vi "Settings Poly.vi"   [LabVIEW 2011]
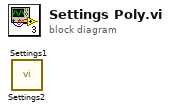
[diagram p0: block diagram]
diagram:
  n1 = call "Settings2.vi"() -> ()  [unwired: 11 in, 1 out]
  n2 = call "Settings1.vi"() -> ()  [unwired: 11 in, 1 out]
